vi "Identity Value.vi"(3 "GUI Identity in":refnum<class "GUI Identity.lvclass">) -> (1 "Value":string)   [LabVIEW 2020, in "VolatusGUI.lvlib" / "GUI Identity.lvclass"]
uses:
  GUI Identity.lvclass
  GUI Identity.lvclass/GUI Identity.ctl
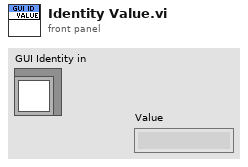
[diagram p1: front panel]
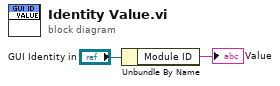
[diagram p0: block diagram]
diagram:
  n1 = Unbundle By Name("GUI Identity in") -> ("Module ID"=→"Value":string)
